vi "launcher.vi"   [LabVIEW 2023]
uses:
  InterferometrUI/InterferometrUI.lvclass
  Applications/National Instruments/LabVIEW 2023 64-bit/vi.lib/ActorFramework/Actor/Actor.lvclass
  <vilib>/ActorFramework/Actor/Actor.lvclass
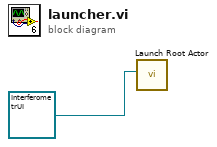
[diagram p0: block diagram]
diagram:
  n1 = call <vilib>:"Launch Root Actor.vi"("Actor"=refnum<class "InterferometrUI.lvclass"> refnum ("InterferometrUI.lvlib:InterferometrUI.lvclass")) -> ()  [unwired: 9 in, 2 out]
